vi "03Foot_GetWave.vi"(11 "Array":u8[](array[numeric])) -> (0 "Waveform 4":i32[](array[numeric]), 1 "Waveform 3":i32[](array[numeric]), 2 "Waveform 2":i32[](array[numeric]), 3 "Waveform 1":i32[](array[numeric]))   [LabVIEW 2015]
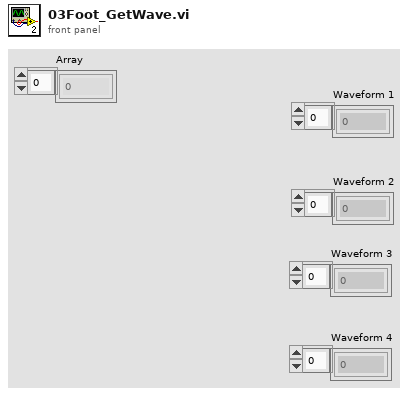
[diagram p1: front panel]
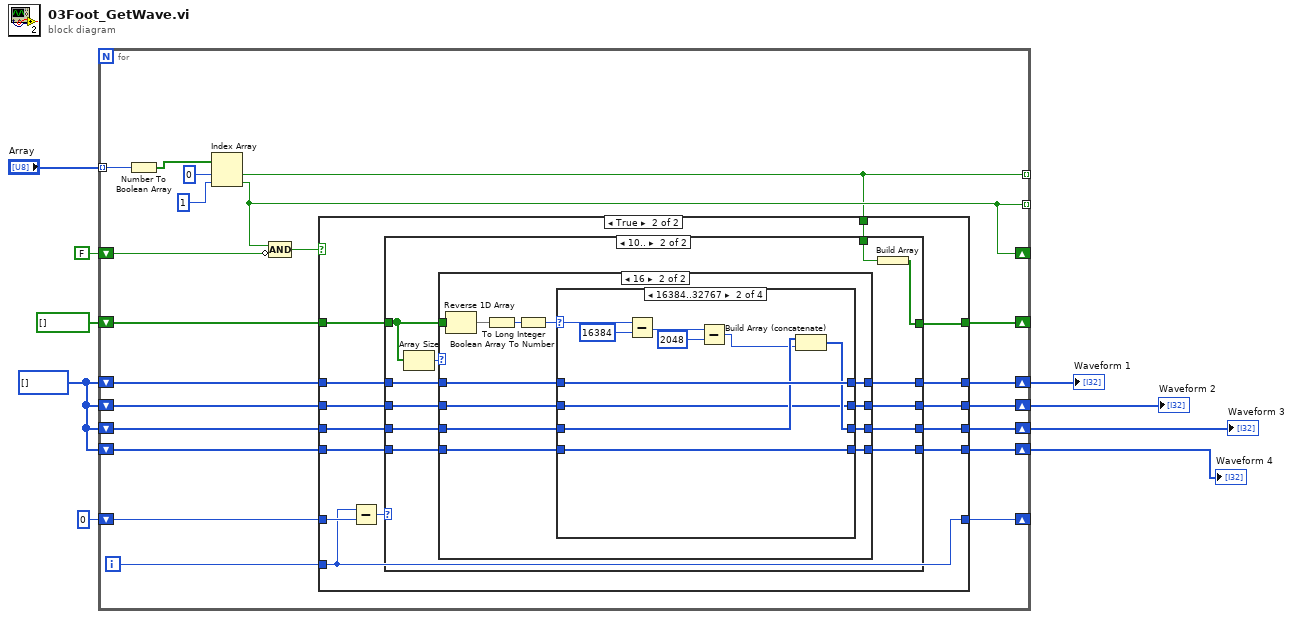
[diagram p0: block diagram]
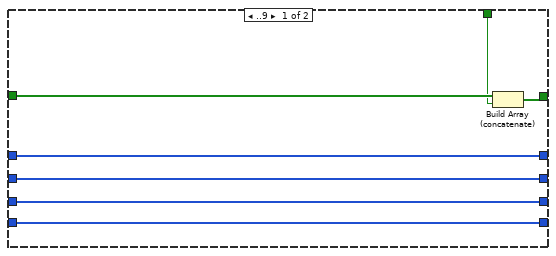
[diagram p3: hidden frame]
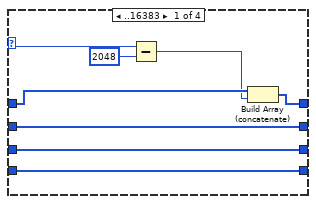
[diagram p5: hidden frame]
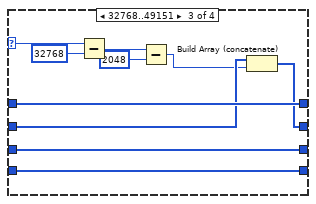
[diagram p6: hidden frame]
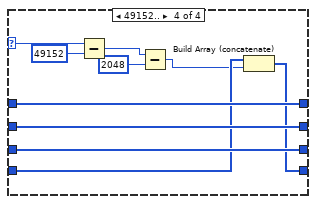
[diagram p7: hidden frame]
diagram:
  w5 = i32[] []
  n1 = for {
    tunnel: "Array" -> [w30] mode=indexing
    tunnel: [w20] -> _ mode=indexing
    tunnel: [w26] -> _ mode=indexing
    shift-right: [w26] -> _
    shift-left: FALSE -> [w25]
    shift-right: [w21] -> _
    shift-left: 0 -> [w22]
    shift-right: [w19] -> _
    shift-left: bool[] [] -> [w18]
    shift-right: [w17] -> w4
    shift-left: w5 -> [w16]
    shift-right: [w12] -> w3
    shift-left: w5 -> [w15]
    shift-right: [w11] -> w2
    shift-left: w5 -> [w14]
    shift-right: [w10] -> w1
    shift-left: w5 -> [w13]
    i -> [w23]
    n2 = Number To Boolean Array(number=w30) -> (Boolean array=w29:bool[])
    n3 = Index Array(array=w29, index #1=0 ("index"), index #2=1 ("index")) -> (element #1=w20:bool, element #2=w26:bool)
    n4 = Compound Arithmetic op=AND(w26, invert w25) -> (w24:bool)
    n5 = case shown="True" w24 {
      tunnel: w23 -> [_ w48]
      tunnel: w22 -> [w36 w50]
      tunnel: [w36 w48] -> w21
      tunnel: w20 -> [_ w47]
      tunnel: [w35 w45] -> w19
      tunnel: w18 -> [w35 w46]
      tunnel: [w34 w43] -> w17
      tunnel: w16 -> [w34 w44]
      tunnel: w15 -> [w33 w42]
      tunnel: w14 -> [w32 w41]
      tunnel: w13 -> [w31 w40]
      tunnel: [w33 w39] -> w12
      tunnel: [w32 w38] -> w11
      tunnel: [w31 w37] -> w10
      frame False {
      }
      frame True {
        n6 = Subtract(x=w48, y=w50) -> (x-y=w49:i32)
        n7 = case shown="10.." w49 {
          tunnel: w47 -> [w56 w68]
          tunnel: w46 -> [w57 w58]
          tunnel: [w55 w69] -> w45
          tunnel: w44 -> [w54 w67]
          tunnel: [w54 w63] -> w43
          tunnel: w42 -> [w53 w66]
          tunnel: w41 -> [w52 w65]
          tunnel: w40 -> [w51 w64]
          tunnel: [w53 w62] -> w39
          tunnel: [w52 w61] -> w38
          tunnel: [w51 w60] -> w37
          frame ..9 {
            n8 = Build Array (concatenate)(w57, w56) -> (w55:bool[])
          }
          frame 10.. {
            n9 = Array Size(array=w58) -> (size(s)=w59:i32)
            n10 = case shown="16" w59 {
              tunnel: w58 -> [_ w85]
              tunnel: w67 -> [w73 w83]
              tunnel: w66 -> [w72 w82]
              tunnel: w65 -> [w71 w81]
              tunnel: w64 -> [w70 w80]
              tunnel: [w73 w79] -> w63
              tunnel: [w72 w78] -> w62
              tunnel: [w71 w77] -> w61
              tunnel: [w70 w76] -> w60
              frame 0, Default {
              }
              frame 16 {
                n11 = Reverse 1D Array(array=w85) -> (reversed array=w84:bool[])
                n12 = Boolean Array To Number(Boolean array=w84) -> (number=w75:u32)
                n13 = To Long Integer(number=w75) -> (32bit integer=w74:i32)
                n14 = case shown="16384..32767" w74 {
                  selector: w74 -> [w88 w101 w111 w122]
                  tunnel: w83 -> [w93 w102 w112 w123]
                  tunnel: w82 -> [w91 w97 w108 w120]
                  tunnel: w81 -> [w90 w99 w109 w119]
                  tunnel: w80 -> [w89 w103 w113 w118]
                  tunnel: [w92 w102 w112 w123] -> w79
                  tunnel: [w91 w97 w107 w120] -> w78
                  tunnel: [w90 w98 w109 w119] -> w77
                  tunnel: [w89 w103 w113 w117] -> w76
                  frame ..16383 {
                    n15 = Subtract(x=w88, y=2048) -> (x-y=w86:i32)
                    n16 = Build Array (concatenate)(w93, w86) -> (w92:i32[])
                  }
                  frame 16384..32767 {
                    n17 = Subtract(x=w101, y=16384) -> (x-y=w96:i32)
                    n18 = Subtract(x=w96, y=2048) -> (x-y=w94:i32)
                    n19 = Build Array (concatenate)(w99, w94) -> (w98:i32[])
                  }
                  frame 32768..49151 {
                    n20 = Subtract(x=w111, y=32768) -> (x-y=w106:i32)
                    n21 = Subtract(x=w106, y=2048) -> (x-y=w104:i32)
                    n22 = Build Array (concatenate)(w108, w104) -> (w107:i32[])
                  }
                  frame 49152.. {
                    n23 = Subtract(x=w122, y=49152) -> (x-y=w116:i32)
                    n24 = Subtract(x=w116, y=2048) -> (x-y=w114:i32)
                    n25 = Build Array (concatenate)(w118, w114) -> (w117:i32[])
                  }
                }
              }
            }
            n26 = Build Array(w68) -> (w69:bool[])
          }
        }
      }
    }
  }
  "Waveform 1" <- w4
  "Waveform 2" <- w3
  "Waveform 3" <- w2
  "Waveform 4" <- w1
